vi "Get_Latest_Dust_Density.vi"(8 "error in (no error)":errorcluster, 11 "Integer Timestamp":dbl) -> (0 "error out":errorcluster, 3 "Density":dbl)   [LabVIEW 2013]
uses:
  <vilib>/addons/database/Connection.llb/Conn Execute.vi
  <vilib>/addons/database/Recordset.llb/Rec Fetch Recordset Data (R).vi
  <vilib>/addons/database/Recordset.llb/Rec Destroy - Connection.vi
  <vilib>/addons/database/_DB Variant To Data/Database Variant To Data.xnode
  <vilib>/addons/database/NI_Database_API.lvlib
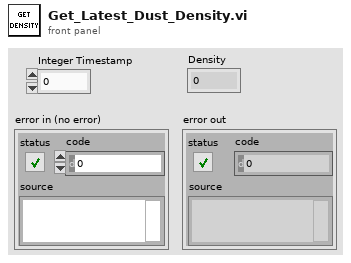
[diagram p1: front panel]
types:
  T1 = typedef "NI_Database_API.lvlib/Conn ObjectReference.ctl" = refnum<k1>
  T2 = typedef "NI_Database_API.lvlib/Rec ObjectReference.ctl" = refnum<k1>
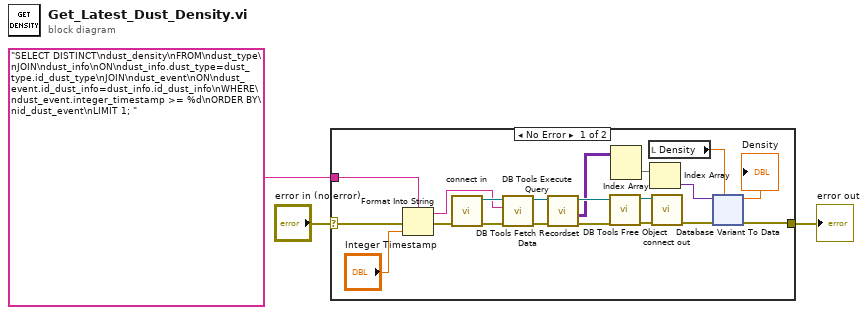
[diagram p0: block diagram]
diagram:
  n1 = case shown="No Error" "error in (no error)" {
    selector: "error in (no error)" -> [w22 w56]
    tunnel: [w4 w56] -> w3
    tunnel: "SELECT DISTINCT\ndust_density\nFROM\ndust_type\nJOIN\ndust_info\nON\ndust_info.dust_type=dust_type.id_dust_type\nJOIN\ndust_event\nON\ndust_event.id_dust_info=dust_info.id_dust_info\nWHERE\ndust_event.integer_timestamp >= %d\nORDER BY\nid_dust_event\nLIMIT 1; " -> [w23 _]
    frame No Error {
      n2 = Format Into String(format string=w23, error in=w22, "Integer Timestamp") -> (resulting string=w17:string, error out=w20:errorcluster)  [unwired: 1 in]
      n3 = call "connect in.vi"("error in (no error)"=w20) -> ("error out"=w19:errorcluster, "Database Connection"=w18:T1)  [unwired: 6 in, 1 out]
      n4 = call-poly <vilib>:"DB Tools Execute Query.vi"("error in (no error)"=w19, "SQL query"=w17, "connection reference"=w18) -> ("error out"=w16:errorcluster, "recordset reference"=w15:T2)  [unwired: 5 in]
      n5 = call-poly <vilib>:"DB Tools Fetch Recordset Data.vi"("error in (no error)"=w16, "recordset reference"=w15) -> ("error out"=w14:errorcluster, "recordset data"=w8:variant[][], "recordset reference out"=w13:T2)  [unwired: 3 in]
      n6 = call-poly <vilib>:"DB Tools Free Object.vi"("error in (no error)"=w14, "recordset reference"=w13) -> ("error out"=w11:errorcluster, "connection reference"=w12:T1)  [unwired: 8 in]
      n7 = Index Array(array=w8) -> (element=w7:variant[])  [unwired: 2 in]
      n8 = local read "Density"() -> (w5:dbl)
      n9 = Index Array(array=w7) -> (element=w6:variant)  [unwired: 1 in]
      n10 = call "connect out.vi"("error in (no error)"=w11, "connection reference"=w12) -> ("error out"=w9:errorcluster)  [unwired: 9 in]
      n11 = xnode "Database Variant To Data"("database variant"=w6, "error in (no error)"=w9, "type"=w5) -> ("data"=→"Density":dbl, "error out"=w4:errorcluster)
    }
    frame Error {
    }
  }
  "error out" <- w3
